vi "Get List of Monkeys in the Process.vi"(8 "error in (no error)":errorcluster, 10 "Process ID":string, 11 "Tamer in":refnum<class "Tamer.lvclass">) -> (0 "error out":errorcluster, 2 "List of Monkeys":string[](array[string]), 3 "Tamer out":refnum<class "Tamer.lvclass">, 4 "Process not found?":bool)   [LabVIEW 2020, in "Tamer.lvlib" / "Tamer.lvclass"]
uses:
  Tamer.lvclass
  Tamer.lvclass/Tamer.ctl
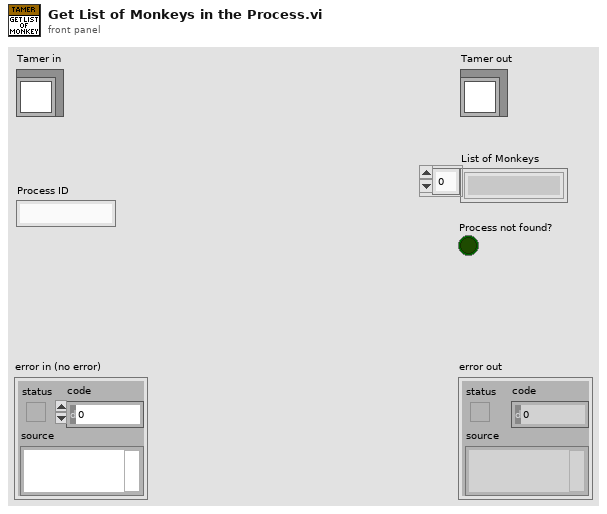
[diagram p1: front panel]
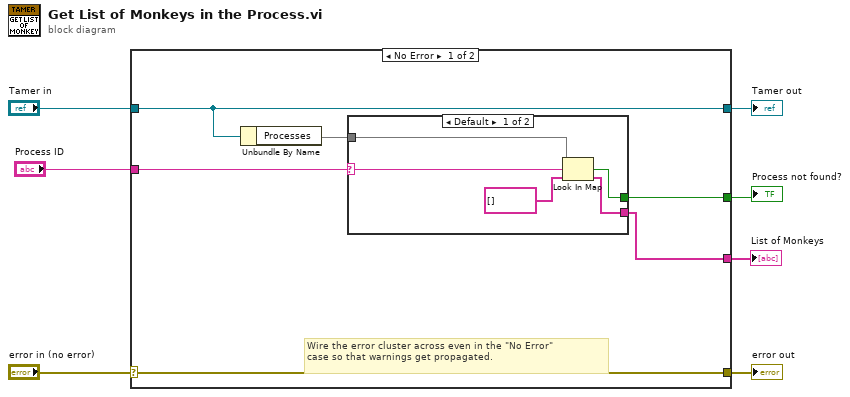
[diagram p0: block diagram]
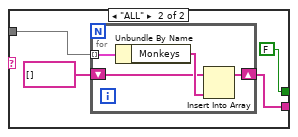
[diagram p2: hidden frame]
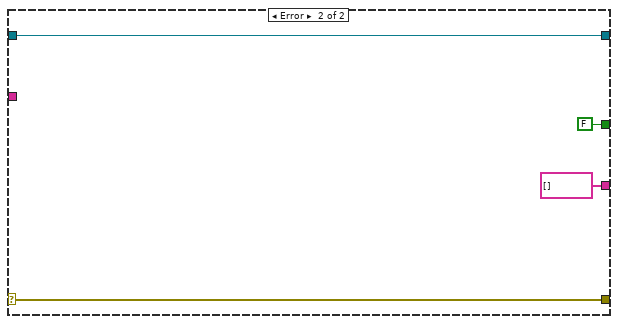
[diagram p3: hidden frame]
diagram:
  n1 = case shown="No Error" "error in (no error)" {
    selector: "error in (no error)" -> [w13 w30]
    tunnel: [w13 w30] -> w6
    tunnel: [w11 w29] -> w4
    tunnel: "Tamer in" -> [w11 w29]
    tunnel: "Process ID" -> [w8 _]
    tunnel: [w10 FALSE ("key not found?")] -> w2
    tunnel: [w9 string[] [] ("array")] -> w1
    frame No Error {
      # "Wire the error cluster across even in the \"No Error\"\ncase so that warnings get propagated."
      n2 = Unbundle By Name(w11) -> ("Processes"=w12:map{string, string[]})
      n3 = case shown="Default" w8 {
        selector: w8 -> [w14 _]
        tunnel: w12 -> [w18 w22]
        tunnel: [w16 w20] -> w9
        tunnel: [w15 FALSE ("key not found?")] -> w10
        frame Default {
          n4 = Look In Map(map=w18, key=w14, default value=string[] []) -> (key not found?=w15:bool, value=w16:string[])
        }
        frame "ALL" {
          n5 = for {
            tunnel: w22 -> [w26] mode=indexing
            shift-right: [w23] -> w20
            shift-left: string[] [] ("array") -> [w24]
            n6 = Unbundle By Name(w26) -> ("Monkeys"=w25:string[])
            n7 = Insert Into Array(array=w24, new element=w25) -> (w23:string[])  [unwired: 1 in]
          }
        }
      }
    }
    frame Error {
    }
  }
  "error out" <- w6
  "Tamer out" <- w4
  "Process not found?" <- w2
  "List of Monkeys" <- w1
